vi "cDAQ Ver 2 Cont Acq Thermocouple Samples-Int Clk-Init.vi"(0 "Physical Channel":tag="cDAQ1Mod1/ai1:15,cDAQ1Mod2/ai0:15,cDAQ1Mod3/ai0:15,cDAQ1Mod4/ai0:15", 1 "Rate":dbl=75.0 format="%0.2f", 3 "error in":errorcluster) -> (7 "Temp task out":refnum<k21>, 10 "error out":errorcluster)   [LabVIEW 2014]
doc: "I. Description:\nThis example demonstrates how to make continuous, hardware-timed temperature measurement using a thermocouple.\n\nII. Instructions for Running:\n1. Specify the Physical Channel where you have connected the thermocouple.\n2. Enter the Minimum and Maximum temperature values in degrees C you expect to measure. A smaller range will allow a more accurate measurement.\n3. Enter the scan rate at which you want to run the acquisition.\n4. Specify the type of thermocouple you are using.\n5. Thermocouple measurements require cold-junction compensation (CJC) to correctly scale them. Specify the source of your cold-junction compensation.\n6. If your CJC source is \"Internal\", skip the rest of the steps.\n7. If your CJC source is \"Constant Value\", specify the value (usually room temperature) in degrees C.\n8. If your CJC source is \"Channel\", specify the CJC Channel name. \n9. Specify the appropriate Auto Zero Mode. See your device's hardware manual to find out if your device supports this attribute.\n\nIII. Block Diagram Steps:\n1. Create a Thermocouple (TC) temperature measurement channel.\n2. Get all the channels in the task.\n3. Convert channel(s) array to a comma-delimited channel string.\n4. This attribute is set to compensate for input offset errors. May not be supported by all devices*.\n5. Call the Timing VI to specify the hardware timing parameters. Use device's internal clock, continuous mode acquisition and the sample rate specified by the user.\n6. Call the Start VI to program and start the acquisition.\n7. Read N samples and plot it. By default, the Read VI reads all available samples, but you can specify how many samples to read at a time and the timeout value. Continue reading data until the stop button is pressed or an error occurs. \n8. Call the Clear Task VI to clear the Task.\n9. Use the popup dialog box to display an error if any.\n\n* If your device does not support Auto Zero Mode bypass Step 2, 3, and 4.\n\nIV. I/O Connections Overview:\nConnect your thermocouple to the terminals corresponding to the Physical Channel I/O Control value."
uses:
  <vilib>/DAQmx/create/channels.llb/DAQmx Create Channel (AI-Temperature-Thermocouple).vi
  <vilib>/DAQmx/configure/timing.llb/DAQmx Timing (Sample Clock).vi
  <vilib>/DAQmx/read.llb/DAQmx Read (Analog 2D DBL NChan NSamp).vi
  <vilib>/Utility/error.llb/DialogType.ctl
  <resource>/objmgr/daqmx.rc
panel:
  in  "Tab Control":enum32{"Page 1", "Page 2"}(tab)
  out "size(s)":i32[](array[numeric])
  out "Array":dbl[](array[numeric])
  in  "number of samples per channel":i32=-1
  out "data":dbl[][](array[numeric]) format="%0.2f"
  out "Numeric":i32
  in  "stop":bool
  out "Measurement":dbl[][](graph)
  # "Timing Parameters"
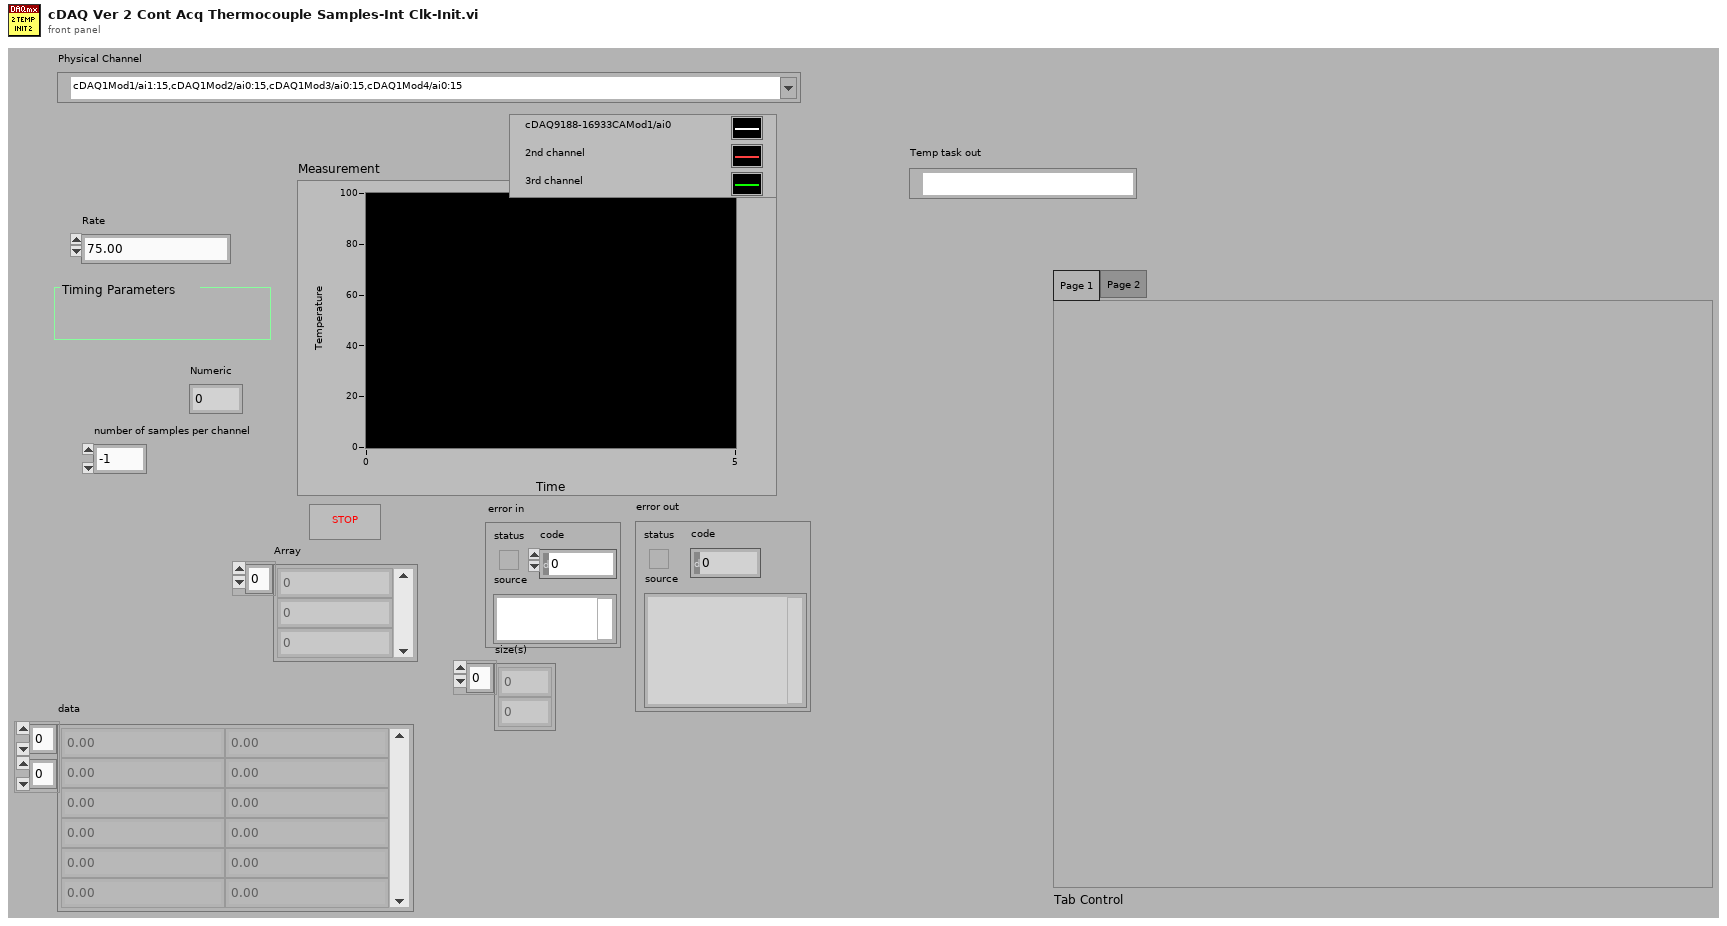
[diagram p1: front panel]
types:
  T1 = typedef "DialogType.ctl" = u16
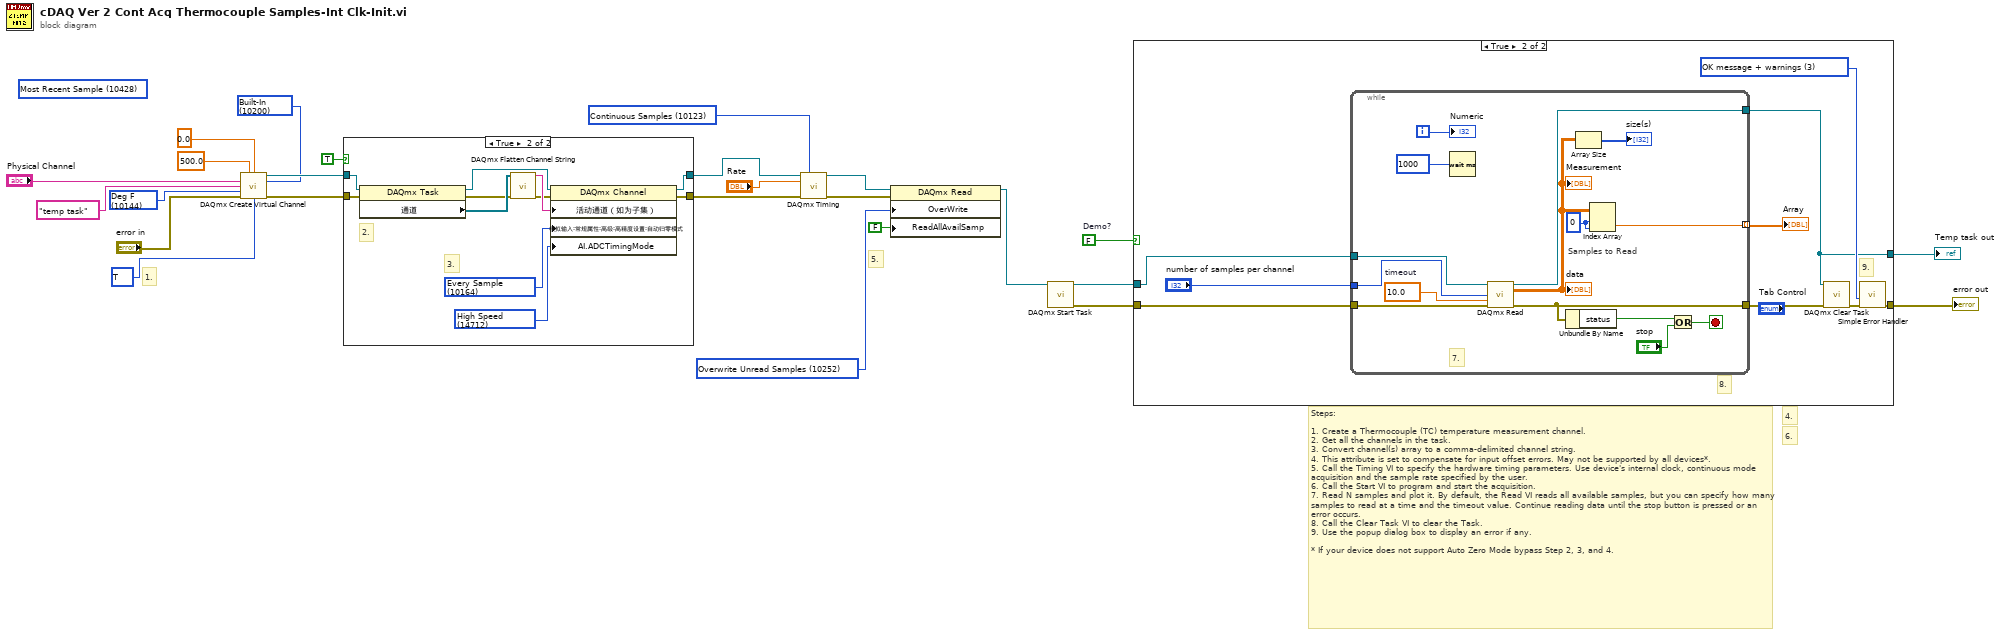
[diagram p0: block diagram]
diagram:
  (unwired) 10428 items=["First Sample"=10424, "Current Read Position"=10425, "Reference Trigger"=10426, "First Pretrigger Sample"=10427, "Most Recent Sample"=10428] ("RelativeTo")
  w17 = 10252 items=["Overwrite Unread Samples"=10252, "Do Not Overwrite Unread Samples"=10159] ("OverWrite")
  w14 = 10144 items=["Deg C"=10143, "Deg F"=10144, "Kelvins"=10325, "Deg R"=10145, "From Custom Scale"=10065] ("units")
  w7 = 10086 items=["J"=10072, "K"=10073, "N"=10077, "R"=10082, "S"=10085, "T"=10086, "B"=10047, "E"=10055] ("Thermocouple Type")
  w13 = 10200 items=["Built-In"=10200, "Constant Value"=10116, "Channel"=10113] ("CJC Source")
  w9 = 10123 items=["Finite Samples"=10178, "Continuous Samples"=10123] ("sample mode")
  w25 = FALSE  # Demo?
  # "5."
  # "1."
  # "4."
  # "6."
  # "Steps: \n\n1. Create a Thermocouple (TC) temperature measurement channel.\n2. Get all the channels in the task.\n3. Convert channel(s) array to a comma-delimited channel string.\n4. This attribute is set to compensate for input offset errors. May not be supported by all devices*.\n5. Call the Timing VI to specify the hardware timing parameters. Use device's internal clock, continuous mode acquisition and the sample rate specified by the user.\n6. Call the Start VI to program and start the acquisition.\n7. Read N samples and plot it. By default, the Read VI reads all available samples, but you can specify how many samples to read at a time and the timeout value. Continue reading data until the stop button is pressed or an error occurs. \n8. Call the Clear Task VI to clear the Task.\n9. Use the popup dialog box to display an error if any.\n\n* If your device does not support Auto Zero Mode bypass Step 2, 3, and 4."
  n1 = call-poly <vilib>:"DAQmx Create Virtual Channel.vi"("maximum value"=500.0 ("Maximum Value (deg C)"), "minimum value"=0.0 ("Minimum Value (degF)"), "physical channels"="Physical Channel", "cjc source"=w13, "name to assign"="temp task", "units"=w14, "error in"="error in", "thermocouple type"=w7) -> ("task out"=w21:refnum<k21>, "error out"=w8:errorcluster)  [unwired: 6 in]
  n2 = case shown="True" TRUE ("SCXI Module?") {
    tunnel: w21 -> [w26 w37]
    tunnel: w8 -> [w27 w36]
    tunnel: [w26 w32] -> w10
    tunnel: [w27 w31] -> w11
    frame False {
      # "Bypass Auto-Zero"
    }
    frame True {
      w28 = 14712 items=["High Resolution"=10195, "High Speed"=14712, "Best 50 Hz Rejection"=14713, "Best 60 Hz Rejection"=14714, "Custom"=10137] ("AI.ADCTimingMode")
      w38 = 10164 items=["None"=10230, "Once"=10244, "Every Sample"=10164] ("Auto Zero Mode")
      # "3."
      # "2."
      n3 = property class="DAQmx Task"(reference=w37, error in=w36) -> (reference out=w35:refnum<k21>, error out=w30:errorcluster, "通道"=w34:refnum<k21>[])
      n4 = call <vilib>:"DAQmx Flatten Channel String.vi"("names in"=w34, "error in"=w30) -> ("names out"=w33:string, "error out"=w29:errorcluster)  [unwired: 12 in]
      n5 = property class="DAQmx Channel"(reference=w35, error in=w29, "活动通道（如为子集）"=w33, "模拟输入:常规属性:高级:高精度设置:自动归零模式"=w38, "AI.ADCTimingMode"=w28) -> (reference out=w32:refnum<k21>, error out=w31:errorcluster)
    }
  }
  n6 = call-poly <vilib>:"DAQmx Timing.vi"("task/channels in"=w10, "sample mode"=w9, "rate"="Rate", "error in"=w11) -> ("task out"=w16:refnum<k21>, "error out"=w18:errorcluster)  [unwired: 10 in]
  n7 = property class="DAQmx Read"(reference=w16, error in=w18, "OverWrite"=w17, "ReadAllAvailSamp"=FALSE) -> (reference out=w3:refnum<k21>)  [unwired: 1 out]
  n8 = call <vilib>:"DAQmx Start Task.vi"("task/channels in"=w3) -> ("task out"=w23:refnum<k21>, "error out"=w24:errorcluster)  [unwired: 13 in]
  n9 = case shown="True" w25 {
    tunnel: w24 -> [w39 w47]
    tunnel: w23 -> [w40 w46]
    tunnel: [w39 w42] -> w4
    tunnel: [w40 w41] -> w2
    frame False {
    }
    frame True {
      w45 = T1 3 items=["no dialog", "OK message", "continue or stop message", "OK message + warnings", "continue/stop + warnings"] ("type of dialog (OK msg:1)")
      # "9."
      # "8."
      n10 = while {
        tunnel: [w61] -> w48
        tunnel: w46 -> [w64]
        tunnel: w47 -> [w63]
        tunnel: [w62] -> w41
        tunnel: "number of samples per channel" -> [w56]
        tunnel: [w53] -> w43 mode=indexing
        i -> [w55]
        stop <- w59 stop-if-true
        w54 = 0 ("index (row)")
        w57 = 10.0  # timeout
        # "Samples to Read"
        # "7."
        n11 = Wait (ms)(milliseconds to wait=u32 1000) -> ()  [unwired: 1 out]
        n12 = call-poly <vilib>:"DAQmx Read.vi"("task/channels in"=w64, "number of samples per channel"=w56, "timeout"=w57, "error in"=w63) -> ("task out"=w62:refnum<k21>, "data"=w52:dbl[][], "error out"=w61:errorcluster)  [unwired: 9 in]
        "Measurement" <- w52
        "data" <- w52
        n13 = Unbundle By Name(w61) -> ("status"=w60:bool)
        n14 = Array Size(array=w52) -> (size(s)=→"size(s)":i32[])
        n15 = Index Array(array=w52, index (row)=w54, index (col)=w54) -> (element=w53:dbl)
        n16 = Or(x=w60, y="stop") -> (x .or. y?=w59:bool)
        "Numeric" <- w55
      }
      "Array" <- w43
      n17 = call <vilib>:"DAQmx Clear Task.vi"("task in"=w41, "error in"=w48) -> ("error out"=w49:errorcluster)  [unwired: 13 in]
      n18 = call <vilib>:"Simple Error Handler.vi"("type of dialog (OK msg:1)"=w45, "error in (no error)"=w49) -> ("error out"=w42:errorcluster)  [unwired: 3 in, 4 out]
    }
  }
  "Temp task out" <- w2
  "error out" <- w4
